vi "Create.vi"(8 "error in (no error)":errorcluster, 11 "minimum log level (Info)":T1=enum."Info") -> (0 "error out":errorcluster, 3 "logger":refnum<class "Logger.lvclass">)   [LabVIEW 2018]
uses:
  src/api/logger_class/Logger.lvclass
  src/api/Log Levels.ctl
  src/api/GLog.lvlib
panel:
  # "Connector Pane"
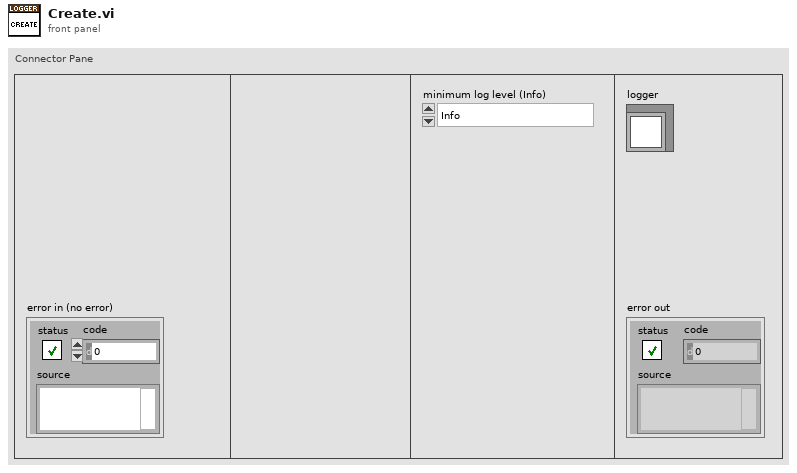
[diagram p1: front panel]
types:
  T1 = typedef "GLog.lvlib/Log Levels.ctl" = enum16{"Trace", "Debug", "Info", "Warning", "Error", "Critical"}
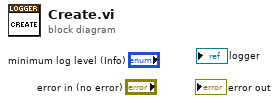
[diagram p0: block diagram]
diagram:
